vi "Drive.vi"() -> ()   [LabVIEW 2012]
uses:
  Robot Global Data.vi
  <vilib>/Rock Robotics/WPI/RobotDrive/WPI_RobotDriveGetSetRefNum.vi
  <vilib>/Rock Robotics/WPI/Joystick/WPI_JoystickGetSetRefNum.vi
  <vilib>/addons/control/pid/NI_PID_pid.lvlib
  <vilib>/addons/control/pid/pid.llb/PID (DBL).vi
panel:
  in  "divide x axis by:":dbl=1.0
  in  "PID gains":T1={"proportional gain (Kc)"=1.0, "integral time (Ti, min)"=0.01, "derivative time (Td, min)"=0.0} {"derivative time (Td, min)" format="%.3f"; "integral time (Ti, min)" format="%.3f"; "proportional gain (Kc)" format="%.3f"}
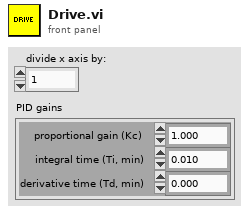
[diagram p1: front panel]
types:
  T1 = cluster{"proportional gain (Kc)":dbl, "integral time (Ti, min)":dbl, "derivative time (Td, min)":dbl}
  T2 = cluster{"Center Position":cluster{"X":dbl, "Y":dbl}, "Distance (ft)":dbl, "Center":bool}[]
  T3 = cluster{"Target Info[0]":cluster{"Center Position":cluster{"X":dbl, "Y":dbl}, "Distance (ft)":dbl, "Center":bool}, "Target Info[1]":cluster{"Center Position":cluster{"X":dbl, "Y":dbl}, "Distance (ft)":dbl, "Center":bool}, "Target Info[2]":cluster{"Center Position":cluster{"X":dbl, "Y":dbl}, "Distance (ft)":dbl, "Center":bool}, "Target Info[3]":cluster{"Center Position":cluster{"X":dbl, "Y":dbl}, "Distance (ft)":dbl, "Center":bool}, "Target Info[4]":cluster{"Center Position":cluster{"X":dbl, "Y":dbl}, "Distance (ft)":dbl, "Center":bool}, "Target Info[5]":cluster{"Center Position":cluster{"X":dbl, "Y":dbl}, "Distance (ft)":dbl, "Center":bool}, "Target Info[6]":cluster{"Center Position":cluster{"X":dbl, "Y":dbl}, "Distance (ft)":dbl, "Center":bool}, "Target Info[7]":cluster{"Center Position":cluster{"X":dbl, "Y":dbl}, "Distance (ft)":dbl, "Center":bool}, "Target Info[8]":cluster{"Center Position":cluster{"X":dbl, "Y":dbl}, "Distance (ft)":dbl, "Center":bool}}
  T4 = cluster{"Center Position":cluster{"X":dbl, "Y":dbl}, "Distance (ft)":dbl, "Center":bool}
  T5 = typedef "WPI_JoystickDevRef.ctl" = cluster{"Device":T6}
  T6 = typedef "WPI_JoystickDeviceEnum.ctl" = enum16{"USB 1", "USB 2", "USB 3", "USB 4", "Kinect 1", "Kinect 2"}
  T7 = typedef "WPI_JoystickButtonState.ctl" = cluster{"Button 1":bool, "Button 2":bool, "Button 3":bool, "Button 4":bool, "Button 5":bool, "Button 6":bool, "Button 7":bool, "Button 8":bool, "Button 9":bool, "Button 10":bool, "Button 11":bool, "Button 12":bool}
  T8 = cluster{"axis 1 (x)":dbl, "axis 2 (y)":dbl, "axis 3 (throttle)":dbl, "axis 4":dbl, "axis 5":dbl, "axis 6":dbl}
  T9 = typedef "WPI_RobotDriveDevRef.ctl" = cluster{"DevStatus":errorcluster, "Motors[]":T10[], "Square Inputs":bool, "Max Output":dbl, "Isochronous":bool}
  T10 = typedef "WPI_MotorControlDeviceRef.ctl" = cluster{"DeviceStatus":errorcluster, "Type":enum16{"PWM", "CAN"}, "PWM":cluster{"Digital Module":T11, "PWM Channel":T12, "DeadBand":T13}, "CAN":cluster{"Device Number":u8, "Control Mode":T14, "Semaphore":T15, "Max Vout":dbl}, "Invert":bool, "TransformRef":T16, "InvTransformRef":T16}
  T11 = typedef "FPGA_TypedefDigitalModule.ctl" = enum16{"Digital Module 1", "Digital Module 2"}
  T12 = typedef "FPGA_DIOPWMChannel.ctl" = enum8{"PWM 1", "PWM 2", "PWM 3", "PWM 4", "PWM 5", "PWM 6", "PWM 7", "PWM 8", "PWM 9", "PWM 10", "Invalid"}
  T13 = typedef "WPI_PWMDeadband.ctl" = cluster{"Name":string, "maxPositivePwm":i32, "minPositivePwm":i32, "centerPwm":i32, "maxNegativePwm":i32, "minNegativePwm":i32, "angularRange":u16}
  T14 = typedef "WPI_CANJaguar_ControlMode.ctl" = enum8{"Percent VBus", "Current", "Speed", "Position", "Voltage"}
  T15 = typedef "Semaphore RefNum" = refnum<k1>
  T16 = typedef "WPI_PWMTransform_ConPane.ctl" = refnum<vi>
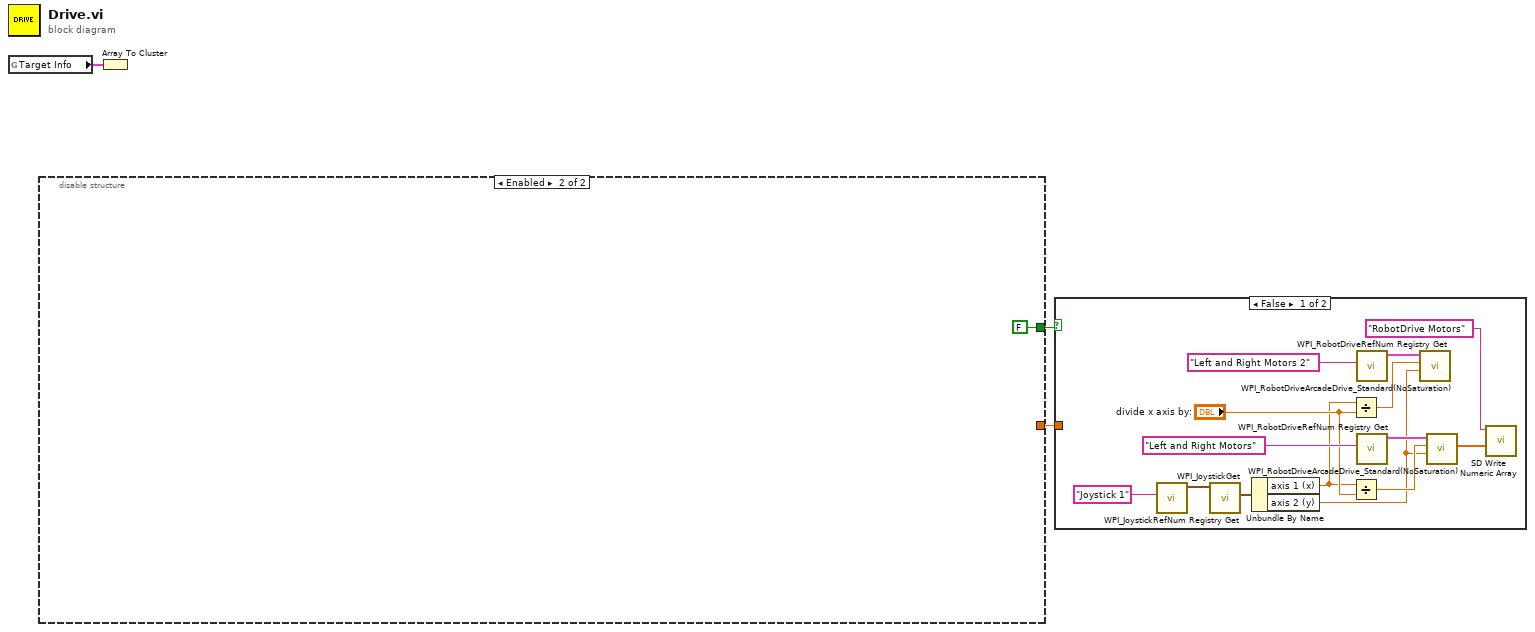
[diagram p0: block diagram]
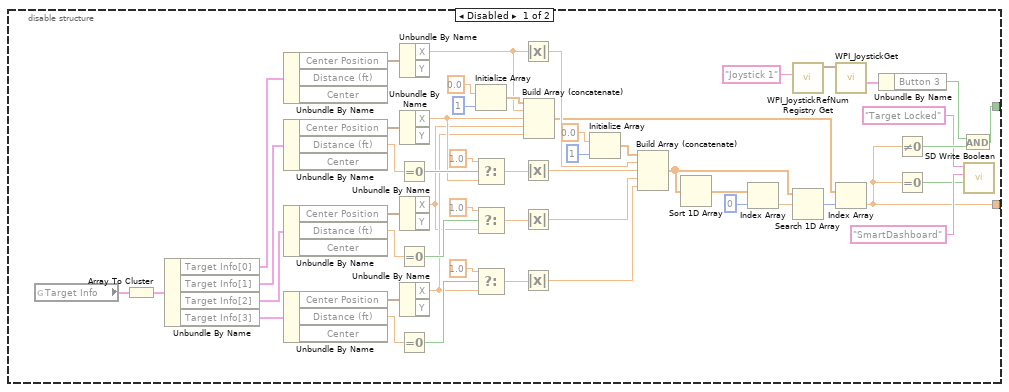
[diagram p2: hidden frame]
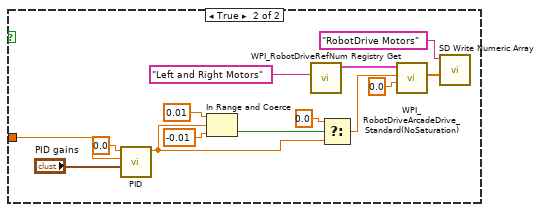
[diagram p3: hidden frame]
diagram:
  n1 = global read "Robot Global Data.vi" "Target Info"() -> (w3:T2)
  n2 = disable-structure shown="Enabled" {
    disable-tunnel: [w7 FALSE] -> w1
    disable-tunnel: [w5 _] -> w2
    frame Disabled {
      n3 = global read "Robot Global Data.vi" "Target Info"() -> (w55:T2)
      n4 = Array To Cluster(array=w55) -> (cluster=w54:T3)
      n5 = Unbundle By Name(w54) -> ("Target Info[0]"=w53:T4, "Target Info[1]"=w48:T4, "Target Info[2]"=w47:T4, "Target Info[3]"=w46:T4)
      n6 = Unbundle By Name(w53) -> ("Center Position"=w52:cluster{"X":dbl, "Y":dbl})  [unwired: 2 out]
      n7 = Unbundle By Name(w48) -> ("Center Position"=w51:cluster{"X":dbl, "Y":dbl}, "Distance (ft)"=w18:dbl)  [unwired: 1 out]
      n8 = Unbundle By Name(w47) -> ("Center Position"=w50:cluster{"X":dbl, "Y":dbl}, "Distance (ft)"=w19:dbl)  [unwired: 1 out]
      n9 = Unbundle By Name(w46) -> ("Center Position"=w49:cluster{"X":dbl, "Y":dbl}, "Distance (ft)"=w20:dbl)  [unwired: 1 out]
      n10 = Equal To 0?(x=w18) -> (x = 0?=w45:bool)
      n11 = Equal To 0?(x=w19) -> (x = 0?=w44:bool)
      n12 = Equal To 0?(x=w20) -> (x = 0?=w43:bool)
      n13 = Unbundle By Name(w52) -> ("X"=w10:dbl)  [unwired: 1 out]
      n14 = Unbundle By Name(w51) -> ("X"=w9:dbl)  [unwired: 1 out]
      n15 = Unbundle By Name(w50) -> ("X"=w6:dbl)  [unwired: 1 out]
      n16 = Unbundle By Name(w49) -> ("X"=w8:dbl)  [unwired: 1 out]
      n17 = Initialize Array(0.0 ("element"), 1 ("dimension size")) -> (w23:dbl[])
      n18 = Select(t=1.0, s=w45, f=w9) -> (s? t:f=w28:dbl)
      n19 = Select(t=1.0, s=w44, f=w6) -> (s? t:f=w27:dbl)
      n20 = Select(t=1.0, s=w43, f=w8) -> (s? t:f=w39:dbl)
      n21 = Absolute Value(x=w10) -> (abs(x)=w35:dbl)
      n22 = Absolute Value(x=w28) -> (abs(x)=w34:dbl)
      n23 = Absolute Value(x=w27) -> (abs(x)=w33:dbl)
      n24 = Absolute Value(x=w39) -> (abs(x)=w26:dbl)
      n25 = Build Array (concatenate)(w23, w10, w9, w6, w8) -> (w22:dbl[])
      n26 = Initialize Array(0.0 ("element"), 1 ("dimension size")) -> (w36:dbl[])
      n27 = Build Array (concatenate)(w36, w35, w34, w33, w26) -> (w29:dbl[])
      n28 = Sort 1D Array(array=w29) -> (sorted array=w32:dbl[])
      n29 = Index Array(array=w32, index=0) -> (element=w30:dbl)
      n30 = call <vilib>:"WPI_JoystickRefNum Registry Get.vi"("refnum name"="Joystick 1") -> ("JoystickDevRef"=w16:T5)  [unwired: 9 in, 1 out]
      n31 = Search 1D Array(1D array=w29, element=w30) -> (index of element=w21:i32)  [unwired: 1 in]
      n32 = call <vilib>:"WPI_JoystickGet.vi"("JoystickDevRef"=w16) -> ("Buttons"=w17:T7)  [unwired: 4 in, 2 out]
      n33 = Index Array(array=w22, index=w21) -> (element=w5:dbl)
      n34 = Unbundle By Name(w17) -> ("Button 3"=w14:bool)
      n35 = Not Equal To 0?(x=w5) -> (x != 0?=w13:bool)
      n36 = Equal To 0?(x=w5) -> (x = 0?=w4:bool)
      n37 = And(x=w14, y=w13) -> (x .and. y?=w7:bool)
      n38 = call <vilib>:"SD Write Boolean.vi"("Boolean"=w4, "Table Prefix"="SmartDashboard", "Name"="Target Locked") -> ()  [unwired: 7 in, 2 out]
    }
    frame Enabled {
    }
  }
  n39 = Array To Cluster(array=w3) -> ()  [unwired: 1 out]
  n40 = case shown="False" w1 {
    tunnel: w2 -> [_ w72]
    frame False {
      n41 = call <vilib>:"WPI_JoystickRefNum Registry Get.vi"("refnum name"="Joystick 1") -> ("JoystickDevRef"=w67:T5)  [unwired: 1 in, 9 out]
      n42 = call <vilib>:"WPI_JoystickGet.vi"("JoystickDevRef"=w67) -> ("Axes"=w66:T8)  [unwired: 1 in, 5 out]
      n43 = Unbundle By Name(w66) -> ("axis 1 (x)"=w57:dbl, "axis 2 (y)"=w59:dbl)
      n44 = Divide(x=w57, y="divide x axis by:") -> (x/y=w58:dbl)
      n45 = Divide(x=w57, y="divide x axis by:") -> (x/y=w63:dbl)
      n46 = call <vilib>:"WPI_RobotDriveRefNum Registry Get.vi"("refnum name"="Left and Right Motors 2") -> ("RobotDriveDevRef"=w62:T9)  [unwired: 1 in, 9 out]
      n47 = call <vilib>:"WPI_RobotDriveRefNum Registry Get.vi"("refnum name"="Left and Right Motors") -> ("RobotDriveDevRef"=w69:T9)  [unwired: 1 in, 9 out]
      n48 = call <vilib>:"WPI_RobotDriveArcadeDrive_Standard(NoSaturation).vi"("Y axis value"=w59, "X axis value"=w58, "RobotDriveDevRef"=w62) -> ()  [unwired: 1 in, 8 out]
      n49 = call <vilib>:"WPI_RobotDriveArcadeDrive_Standard(NoSaturation).vi"("Y axis value"=w59, "X axis value"=w63, "RobotDriveDevRef"=w69) -> ("Motor Values"=w64:dbl[])  [unwired: 1 in, 7 out]
      n50 = call <vilib>:"SD Write Numeric Array.vi"("Numeric Array"=w64, "Name"="RobotDrive Motors") -> ()  [unwired: 8 in, 2 out]
    }
    frame True {
      n51 = call-poly <vilib>:"PID.vi"("PID gains"="PID gains", "process variable"=w72, "setpoint"=0.0 ("process variable")) -> ("output"=w73:dbl)  [unwired: 7 in, 1 out]
      n52 = In Range and Coerce(upper limit=0.01, x=w73, lower limit=-0.01) -> (In Range?=w75:bool)  [unwired: 1 out]
      n53 = call <vilib>:"WPI_RobotDriveRefNum Registry Get.vi"("refnum name"="Left and Right Motors") -> ("RobotDriveDevRef"=w81:T9)  [unwired: 1 in, 9 out]
      n54 = Select(t=0.0, s=w75, f=w73) -> (s? t:f=w71:dbl)
      n55 = call <vilib>:"WPI_RobotDriveArcadeDrive_Standard(NoSaturation).vi"("Y axis value"=0.0, "X axis value"=w71, "RobotDriveDevRef"=w81) -> ("Motor Values"=w80:dbl[])  [unwired: 1 in, 7 out]
      n56 = call <vilib>:"SD Write Numeric Array.vi"("Numeric Array"=w80, "Name"="RobotDrive Motors") -> ()  [unwired: 8 in, 2 out]
    }
  }
